vi "GetStringIndex.vi"(8 "Error In":errorcluster, 10 "Colum Index":u16, 11 "Row Index":u16) -> (0 "error IO":errorcluster, 2 "Colum Index":string, 3 "Row Index":string)   [LabVIEW 2016]
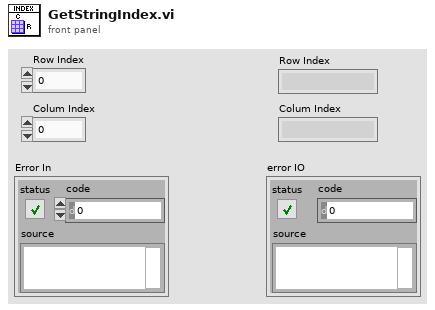
[diagram p1: front panel]
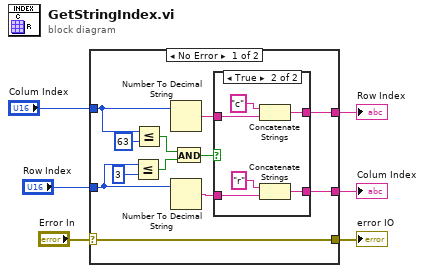
[diagram p0: block diagram]
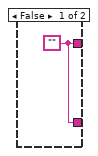
[diagram p2: hidden frame]
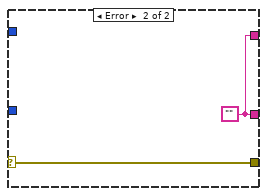
[diagram p3: hidden frame]
diagram:
  n1 = case shown="No Error" "Error In" {
    selector: "Error In" -> [w9 w26]
    tunnel: "Colum Index" -> [w10 _]
    tunnel: "Row Index" -> [w12 _]
    tunnel: [w18 w27] -> w2
    tunnel: [w17 w27] -> w1
    tunnel: [w9 w26] -> w3
    frame No Error {
      n2 = Less Or Equal?(x=w12, y=u16 3) -> (x <= y?=w8:bool)
      n3 = Less Or Equal?(x=w10, y=u16 63) -> (x <= y?=w7:bool)
      n4 = Number To Decimal String(number=w10) -> (decimal integer string=w11:string)  [unwired: 1 in]
      n5 = Number To Decimal String(number=w12) -> (decimal integer string=w13:string)  [unwired: 1 in]
      n6 = And(x=w7, y=w8) -> (x .and. y?=w14:bool)
      n7 = case shown="True" w14 {
        tunnel: [w19 w23] -> w18
        tunnel: [w19 w22] -> w17
        tunnel: w13 -> [_ w21]
        tunnel: w11 -> [_ w20]
        frame False {
          w19 = ""
        }
        frame True {
          n8 = Concatenate Strings("c" ("string"), w20) -> (w23:string)
          n9 = Concatenate Strings("r" ("string"), w21) -> (w22:string)
        }
      }
    }
    frame Error {
      w27 = ""
    }
  }
  "error IO" <- w3
  "Row Index" <- w2
  "Colum Index" <- w1
